vi "Delete DUT Connector Band.vi"(4 "Bands":cluster{"Type (LTE)":i32, "Band Number":i32}[](array[cluster]) {"Type (LTE)" items=["LTE", "New Radio", "WLAN"]}, 6 "RX (RX0)":i32(ring) items=["RX0", "RX1", "RX2", "RX3", "None"], 7 "TX (TX0)":i32(ring) items=["TX0", "TX1", "None"], 8 "error in (no error)":errorcluster, 9 "Connector (\"Connector1\")":string="Connector1", 10 "DUT (\"DUT1\")":string="DUT1", 11 "VISA resource name":refnum<visa-resource-name>) -> (0 "error out":errorcluster, 3 "VISA resource name out":refnum<visa-resource-name>)   [LabVIEW 2015, in "Rohde&Schwarz CMXP Base.lvlib"]
doc: "Removes frequency bands from an antenna connector of the inactive DUT (connector-centric approach).\n\nYou can remove several bands. Specify the technology and the band number for each band.\n\nAttribute:\n-\n\nRemote-control command:\nREMove:DUT:PROFile:CONNector:BAND"
uses:
  <instrlib>/Rohde&Schwarz CMXP Base/Rohde&Schwarz CMXP Base.lvlib
  <instrlib>/Rohde&Schwarz CMXP Base/Private/rsidr_core.llb/rsidr_core.lvlib
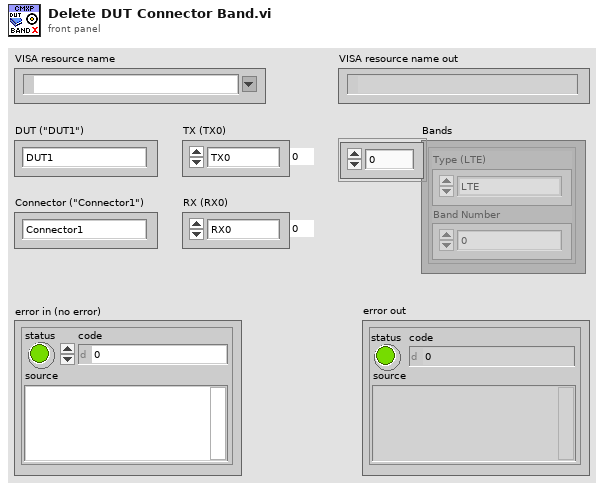
[diagram p1: front panel]
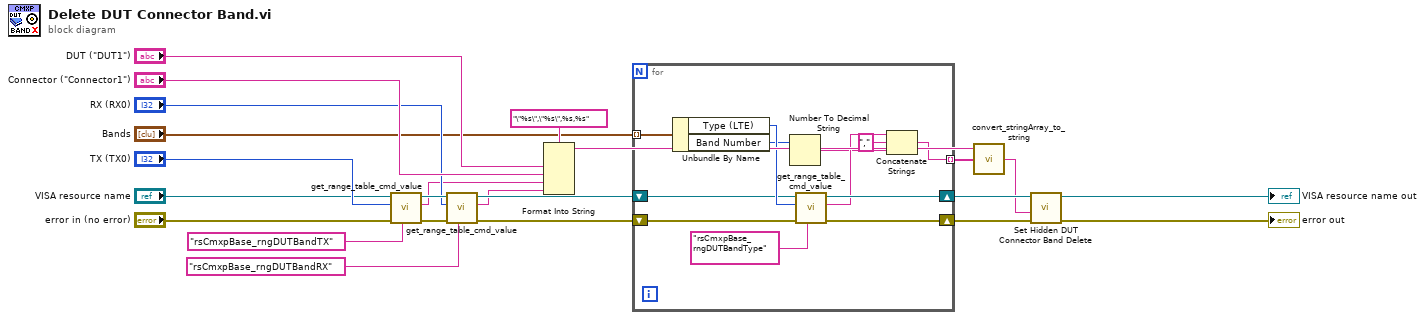
[diagram p0: block diagram]
diagram:
  n1 = call <instrlib>:"get_range_table_cmd_value.vi"("Range Table ID in"="rsCmxpBase_rngDUTBandTX", "error in"="error in (no error)", "Input Int32 value"="TX (TX0)", "VISA resource name"="VISA resource name") -> ("error out"=w22:errorcluster, "Cmd value out"=w3:string, "VISA resource name out"=w23:refnum<visa-resource-name>)  [unwired: 5 in]
  n2 = call <instrlib>:"get_range_table_cmd_value.vi"("Range Table ID in"="rsCmxpBase_rngDUTBandRX", "error in"=w22, "Input Int32 value"="RX (RX0)", "VISA resource name"=w23) -> ("error out"=w8:errorcluster, "Cmd value out"=w2:string, "VISA resource name out"=w7:refnum<visa-resource-name>)  [unwired: 5 in]
  n3 = Format Into String(format string="\"%s\",\"%s\",%s,%s", "DUT (\"DUT1\")", "Connector (\"Connector1\")", w3, w2) -> (resulting string=w9:string)  [unwired: 2 in, 1 out]
  n4 = for {
    tunnel: "Bands" -> [w35] mode=indexing
    tunnel: [w28] -> w10 mode=indexing
    shift-right: [w30] -> w4
    shift-left: w7 -> [w32]
    shift-right: [w29] -> w5
    shift-left: w8 -> [w34]
    n5 = Unbundle By Name(w35) -> ("Type (LTE)"=w33:i32, "Band Number"=w25:i32)
    n6 = Number To Decimal String(number=w25) -> (decimal integer string=w24:string)  [unwired: 1 in]
    n7 = call <instrlib>:"get_range_table_cmd_value.vi"("Range Table ID in"="rsCmxpBase_rngDUTBandType", "error in"=w34, "Input Int32 value"=w33, "VISA resource name"=w32) -> ("error out"=w29:errorcluster, "Cmd value out"=w27:string, "VISA resource name out"=w30:refnum<visa-resource-name>)  [unwired: 5 in]
    n8 = Concatenate Strings(w27, "," ("string"), w24) -> (w28:string)
  }
  n9 = call <instrlib>:"convert_stringArray_to_string.vi"("string array in"=w10, "String to add before (\"\")"=w9) -> ("string out"=w1:string)  [unwired: 3 in]
  n10 = call "Set Hidden DUT Connector Band Delete"("error in (no error)"=w5, "Hidden DUT Connector Band Delete ()"=w1, "instrument handle"=w4) -> ("error out"=→"error out":errorcluster, "instrument handle out"=→"VISA resource name out":refnum<visa-resource-name>)  [unwired: 7 in]
